vi "SENS_SEGM_BWID_RES.vi"(0 "VISA IN":refnum<visa-resource-name>, 1 "Segment":i32, 2 "IF BW(Hz)":i32, 5 "error in":errorcluster, 7 "Channel":i32) -> (14 "VISA Out":refnum<visa-resource-name>, 19 "error out":errorcluster)   [LabVIEW 2018, in "PNA-X.lvlib"]
doc: "SENSe<cnum>:SEGMent<snum>:BWIDth[:RESolution] <num> \n(Read-Write) Sets the IF Bandwidth for the specified segment. First set \nSENS:SEGM:BWIDth:CONTrol ON. All subsequent segments that are added assume the \nnew IF Bandwidth value. \nParameters \n<cnum> Any existing channel number. If unspecified, value is set to 1 \n<snum> Segment number to modify. Choose any existing segment number. \n<num> IF Bandwidth in Hz. The list of valid IF Bandwidths is different depending on \nthe PNA model. (Click to see the lists.) If an invalid number is specified, the \nanalyzer will round up to the closest valid number. \nNote: This command will accept MIN or MAX instead of a numeric parameter. \nSee SCPI Syntax for more information. \nExamples SENS:SEGM:BWID 1KHZ \nsense2:segment2:bwidth:resolution max \nQuery Syntax SENSe<cnum>:SEGMent<snum>:BWIDth[:RESolution]? \nReturn Type Numeric \nDefault See Preset IFBW for your PNA model."
uses:
  PNA-X.lvlib
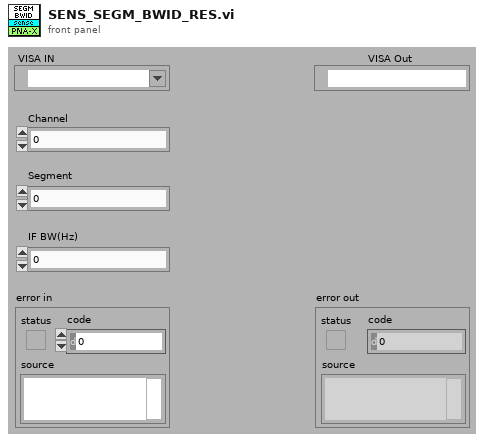
[diagram p1: front panel]
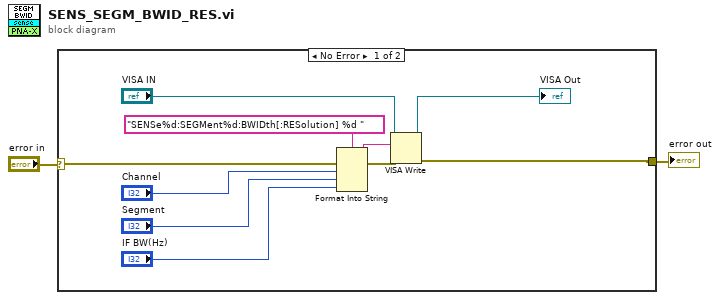
[diagram p0: block diagram]
diagram:
  n1 = case shown="No Error" "error in" {
    selector: "error in" -> [w12 w13]
    tunnel: [w7 w13] -> w1
    frame No Error {
      n2 = Format Into String(format string="SENSe%d:SEGMent%d:BWIDth[:RESolution] %d " ("Cmdline"), error in=w12, "Channel", "Segment", "IF BW(Hz)") -> (resulting string=w10:string, error out=w11:errorcluster)  [unwired: 1 in]
      n3 = VISA Write(VISA resource name="VISA IN", write buffer=w10, error in (no error)=w11) -> (VISA resource name out=→"VISA Out":refnum<visa-resource-name>, error out=w7:errorcluster)  [unwired: 1 out]
    }
    frame Error {
    }
  }
  "error out" <- w1
